vi "clone.vi"(0 "reference":refnum<class "NoteNode.lvclass">, 5 "error in (no error)":errorcluster) -> (14 "reference out":refnum<class "NoteNode.lvclass">, 15 "clonedNote":refnum<class "AbstractNode.lvclass">, 19 "error out":errorcluster)   [LabVIEW 2014, in "NoteNode.lvclass"]
doc: "public Object clone()"
uses:
  <resource>/Framework/Providers/Open_GDS/UML/NoteNode_class/NoteNode.lvclass
  <resource>/Framework/Providers/Open_GDS/UML/AbstractNode_class/AbstractNode.lvclass
  <resource>/Framework/Providers/Open_GDS/UML/MultiLineString_class/MultiLineString.lvclass
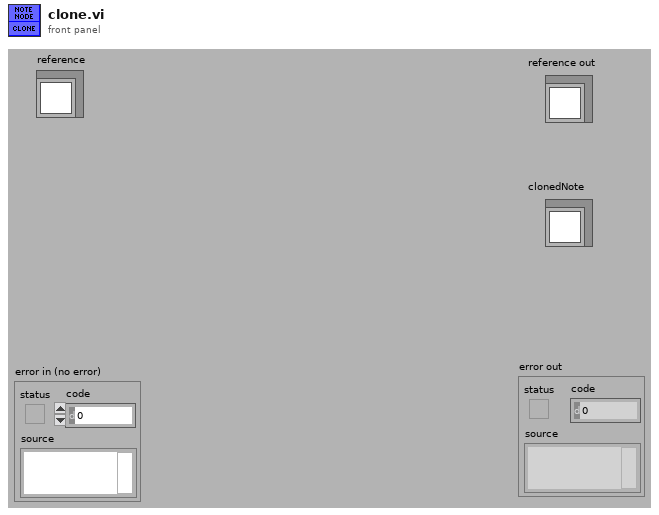
[diagram p1: front panel]
types:
  T1 = typedef "NoteNode.lvclass/ObjectAttributes.ctl" = cluster{"DEFAULT_WIDTH":i32, "DEFAULT_HEIGHT":i32, "DEFAULT_COLOR":u32, "FOLD_X":i32, "FOLD_Y":i32, "color":u32, "text":refnum<class "MultiLineString.lvclass">, "pointNodes":refnum<class "AbstractNode.lvclass">[]}
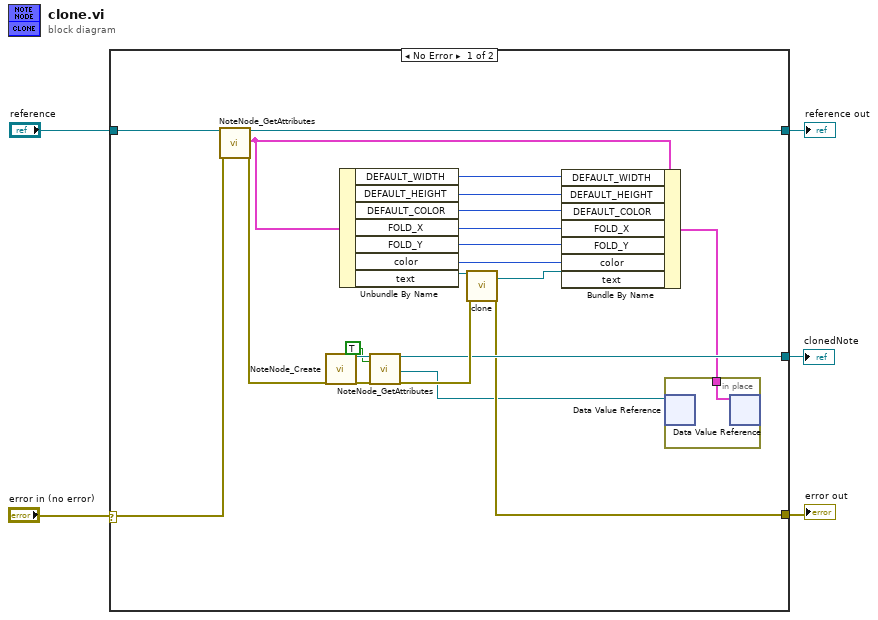
[diagram p0: block diagram]
diagram:
  n1 = case shown="No Error" "error in (no error)" {
    selector: "error in (no error)" -> [w24 w28]
    tunnel: "reference" -> [w26 w29]
    tunnel: [w8 w28] -> w4
    tunnel: [w25 w29] -> w3
    tunnel: [w9 _] -> w1
    frame No Error {
      n2 = call <resource>:"NoteNode_GetAttributes.vi"("reference in"=w26, "error in (no error)"=w24) -> ("reference out"=w25:refnum<class "NoteNode.lvclass">, "Data"=w10:T1, "error out"=w12:errorcluster)  [unwired: 1 in, 14 out]
      n3 = call <resource>:"NoteNode_Create.vi"("error in (no error)"=w12) -> ("reference out"=w13:refnum<class "NoteNode.lvclass">, "error out"=w23:errorcluster)  [unwired: 17 in]
      n4 = Unbundle By Name(w10) -> ("DEFAULT_WIDTH"=w22:i32, "DEFAULT_HEIGHT"=w21:i32, "DEFAULT_COLOR"=w20:u32, "FOLD_X"=w19:i32, "FOLD_Y"=w18:i32, "color"=w14:u32, "text"=w17:refnum<class "MultiLineString.lvclass">)
      n5 = call <resource>:"NoteNode_GetAttributes.vi"("reference in"=w13, "OnlyGetDvrReference(False)"=TRUE, "error in (no error)"=w23) -> ("reference out"=w9:refnum<class "NoteNode.lvclass">, "DataRef"=w7:refnum<data-value>, "error out"=w16:errorcluster)  [unwired: 13 in, 1 out]
      n6 = call-dynamic "clone.vi"("reference"=w17, "error in (no error)"=w16) -> ("clonedMultiLineString"=w15:refnum<class "MultiLineString.lvclass">, "error out"=w8:errorcluster)  [unwired: 15 in, 1 out]
      n7 = Bundle By Name(cluster=w10, "DEFAULT_WIDTH"=w22, "DEFAULT_HEIGHT"=w21, "DEFAULT_COLOR"=w20, "FOLD_X"=w19, "FOLD_Y"=w18, "color"=w14, "text"=w15) -> (w6:T1)
      n8 = in-place {
        in-place-border: w6 -> [w27]
        n9 = in-place-dvr #1(w7) -> ()  [unwired: 2 out]
        n10 = in-place-dvr #1(w27) -> ()  [unwired: 2 out]
      }
    }
    frame Error {
    }
  }
  "reference out" <- w3
  "error out" <- w4
  "clonedNote" <- w1
